vi "New Panel Launched.vi"(8 "error in (no error)":errorcluster, 9 "Name":string, 10 "VI Refnum":refnum<vi>, 11 "Chat Window Model in":refnum<class "Chat Window Model.lvclass">) -> (0 "error out":errorcluster, 3 "Chat Window Model out":refnum<class "Chat Window Model.lvclass">)   [LabVIEW 2014, in "Chat Window Model.lvlib" / "Chat Window Model.lvclass"]
uses:
  Chat Window Model.lvclass
  Chat Window Model Messages/New UI Reference Msg/New UI Reference Msg.lvclass
  <vilib>/ActorFramework/Actor/Actor.lvclass
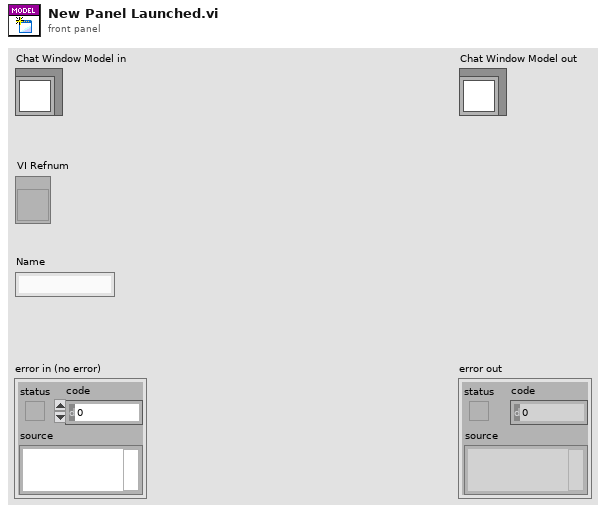
[diagram p1: front panel]
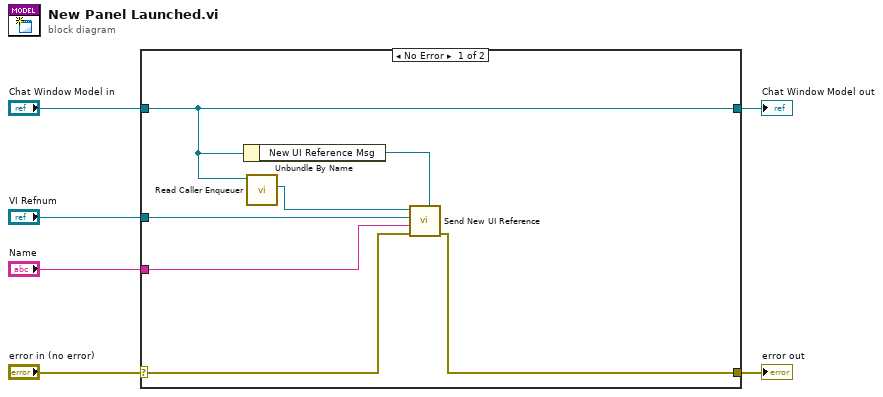
[diagram p0: block diagram]
diagram:
  n1 = case shown="No Error" "error in (no error)" {
    selector: "error in (no error)" -> [w10 w15]
    tunnel: [w9 w15] -> w5
    tunnel: [w8 w14] -> w3
    tunnel: "Chat Window Model in" -> [w8 w14]
    tunnel: "VI Refnum" -> [w12 _]
    tunnel: "Name" -> [w11 _]
    frame No Error {
      n2 = Unbundle By Name(w8) -> ("New UI Reference Msg"=w13:refnum<class "New UI Reference Msg.lvclass">)
      n3 = call <vilib>:"Read Caller Enqueuer.vi"("Actor"=w8) -> ("Caller Enqueuer"=w7:refnum<class "Message Enqueuer.lvclass">)  [unwired: 10 in]
      n4 = call "Send New UI Reference.vi"("Message Type"=w13, "error in (no error)"=w10, "Name"=w11, "VI Refnum"=w12, "Message Enqueuer"=w7) -> ("error out"=w9:errorcluster)  [unwired: 5 in, 1 out]
    }
    frame Error {
    }
  }
  "error out" <- w5
  "Chat Window Model out" <- w3
